vi "Win32 WriteConsole.vi"(8 "error in (no error)":errorcluster, 11 "StdOut":string) -> (0 "error out":errorcluster, 1 "Has Console?":bool)   [LabVIEW 2018, in "Pkg.lvlib"]
uses:
  Pkg.lvlib
  Kernel32.dll
  <vilib>/ErrorRing/Error Ring.xnode
  <vilib>/Utility/error.llb/Error Cluster From Error Code.vi
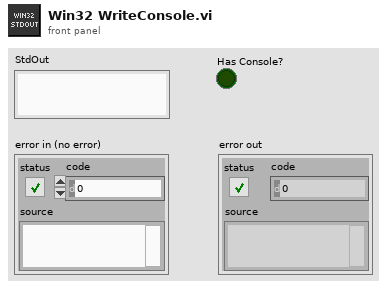
[diagram p1: front panel]
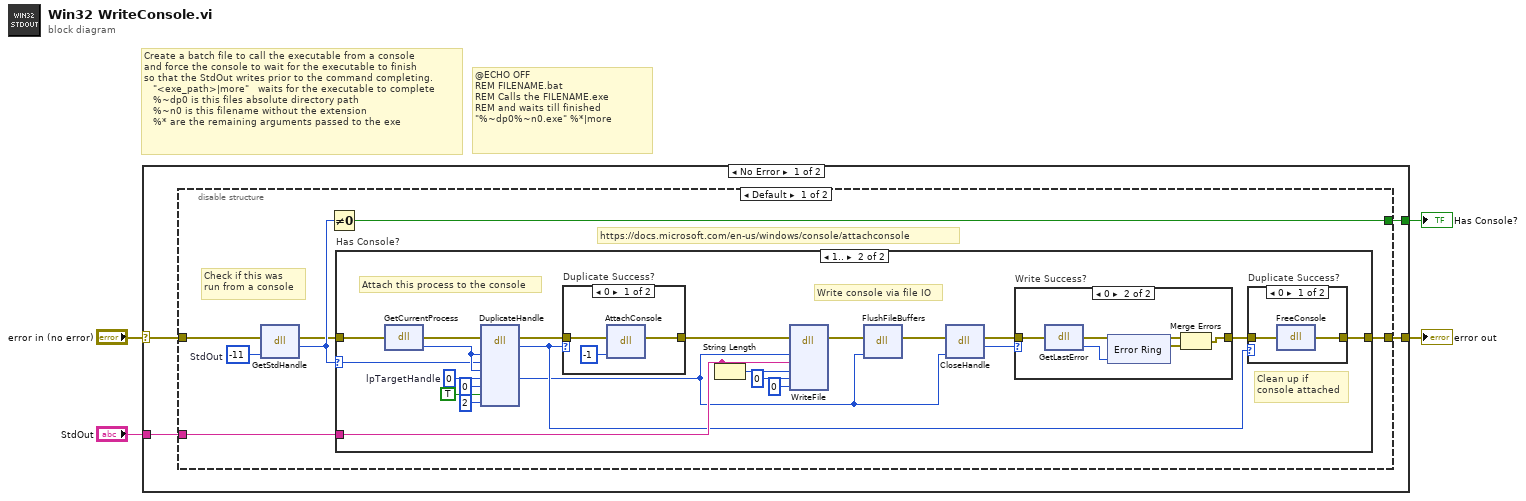
[diagram p0: block diagram]
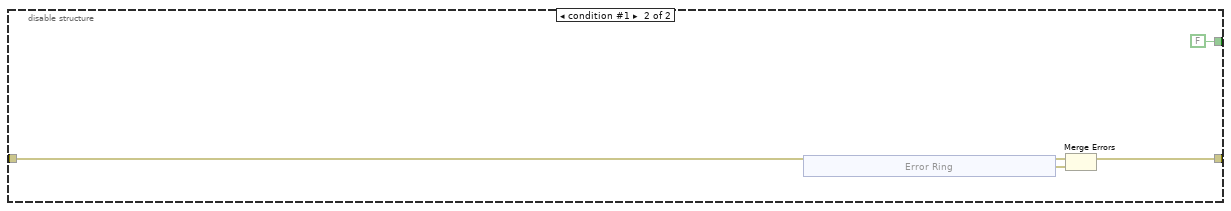
[diagram p6: hidden frame]
diagram:
  # "Create a batch file to call the executable from a console \nand force the console to wait for the executable to finish\nso that the StdOut writes prior to the command completing.\n   \"<exe_path>|more\"   waits for the executable to complete\n   %~dp0 is this files absolute directory path\n   %~n0 is this filename without the extension\n   %* are the remaining arguments passed to the exe"
  # "@ECHO OFF\nREM FILENAME.bat\nREM Calls the FILENAME.exe\nREM and waits till finished\n\"%~dp0%~n0.exe\" %*|more"
  n1 = case shown="No Error" "error in (no error)" {
    selector: "error in (no error)" -> [w6 w67]
    tunnel: [w8 w67] -> w4
    tunnel: [w7 _] -> w3
    tunnel: "StdOut" -> [w5 _]
    frame No Error {
      n2 = disable-structure shown="Default" {
        disable-tunnel: [w14 w61] -> w8
        disable-tunnel: [w12 FALSE] -> w7
        disable-tunnel: w6 -> [w10 w60]
        disable-tunnel: w5 -> [w9 _]
        frame condition #0 (active) {
          w15 = -11  # StdOut
          # "https://docs.microsoft.com/en-us/windows/console/attachconsole"
          # "Check if this was\nrun from a console"
          n3 = dll-call lib="kernel32.dll" fn="GetStdHandle"(error in=w10, "nStdHandle"=w15) -> (error out=w11:errorcluster, "return type"=w13:u64)  [unwired: 3 in, 1 out]
          n4 = Not Equal To 0?(x=w13) -> (x != 0?=w12:bool)
          n5 = case "Has Console?" shown="1.." w13 {
            selector: w13 -> [_ w27]
            tunnel: [w16 w32] -> w14
            tunnel: w11 -> [w16 w31]
            tunnel: w9 -> [_ w29]
            frame 0 {
            }
            frame 1.. {
              w28 = u64 0  # lpTargetHandle
              # "Clean up if \nconsole attached"
              # "Write console via file IO"
              # "Attach this process to the console"
              n6 = dll-call lib="kernel32.dll" fn="GetCurrentProcess"(error in=w31) -> (error out=w30:errorcluster, "return type"=w38:u64)  [unwired: 2 in, 1 out]
              n7 = dll-call lib="kernel32.dll" fn="DuplicateHandle"(error in=w30, "hSourceProcess"=w38, "hSourceHandle"=w27, "hTargetProcess"=w38, "lpTargetHandle"=w28, "dwDesirecAccess"=u16 0, "bInheritHandle"=TRUE, "dwOptions"=u16 2) -> (error out=w37:errorcluster, "return type"=w26:i32, "lpTargetHandle"=w17:u64)  [unwired: 8 in, 1 out]
              n8 = case "Duplicate Success?" shown="0" w26 {
                tunnel: w37 -> [w41 w42]
                tunnel: [w40 w42] -> w25
                frame 0 {
                  n9 = dll-call lib="kernel32.dll" fn="AttachConsole"(error in=w41, "dwProcessId"=-1 ("arg1")) -> (error out=w40:errorcluster)  [unwired: 4 in, 1 out]
                }
                frame Default {
                  # "Duplicated"
                }
              }
              n10 = String Length(string=w29) -> (length=w22:i32)
              n11 = dll-call lib="kernel32.dll" fn="WriteFile"(error in=w25, "hFile"=w17, "lpBuffer"=w29, "nNumberOfBytesToWrite"=w22, "lpNumberofBytesWritten"=0, "lpOverlapped"=u64 0) -> (error out=w24:errorcluster)  [unwired: 7 in, 2 out]
              n12 = dll-call lib="kernel32.dll" fn="FlushFileBuffers"(error in=w24, "hFile"=w17) -> (error out=w23:errorcluster)  [unwired: 3 in, 2 out]
              n13 = dll-call lib="kernel32.dll" fn="CloseHandle"(error in=w23, "nStdHandle"=w17) -> (error out=w21:errorcluster, "return type"=w20:i32)  [unwired: 3 in, 1 out]
              n14 = case "Write Success?" shown="0" w20 {
                tunnel: w21 -> [w43 w48]
                tunnel: [w43 w46] -> w33
                frame Default {
                  # "Closed"
                }
                frame 0 {
                  n15 = dll-call lib="kernel32.dll" fn="GetLastError"(error in=w48) -> (error out=w47:errorcluster, "return type"=w44:i32)  [unwired: 2 in, 1 out]
                  n16 = xnode "Error Ring"("parameter 0"=w44) -> ("error out"=w45:errorcluster)
                  n17 = Merge Errors(w47, w45) -> (w46:errorcluster)
                }
              }
              n18 = case "Duplicate Success?" shown="0" w26 {
                tunnel: w33 -> [w57 w58]
                tunnel: [w56 w58] -> w32
                frame 0 {
                  n19 = dll-call lib="kernel32.dll" fn="FreeConsole"(error in=w57) -> (error out=w56:errorcluster)  [unwired: 2 in, 2 out]
                }
                frame Default {
                  # "Duplicated"
                }
              }
            }
          }
        }
        frame condition #1 {
          n20 = xnode "Error Ring"() -> ("error out"=w62:errorcluster)
          n21 = Merge Errors(w60, w62) -> (w61:errorcluster)
        }
      }
    }
    frame Error {
    }
  }
  "error out" <- w4
  "Has Console?" <- w3
